vi "SerialRPC.vi"(8 "error in (no error)":errorcluster, 9 "Timeout":dbl=10000.0, 10 "Serial Port":refnum<visa-resource-name>="COM5", 11 "Baud Rate":u32=9600) -> (0 "error out":errorcluster, 3 "mbed.lvclass":refnum<class "mbed.lvclass">)   [LabVIEW 2011, in "mbed_LVLibrary.lvlib" / "SerialRPC.lvclass"]
doc: "This constructs an mbed object connected over Serial port. The mbed must be running code which receives data over the USB virtual serial port and passes it to the RPC function. See the mbed cookbook for code for the mbed http://mbed.org/cookbook/Interfacing-with-LabVIEW \nPass into this the port and baud rate."
uses:
  SerialRPC.lvclass
  mbed/mbed.lvclass
  <vilib>/Instr/_visa.llb/VISA Set IO Buffer Mask.ctl
  SerialRPC.lvclass/SerialRPC.ctl
  <vilib>/Instr/_visa.llb/VISA Configure Serial Port (Instr).vi
panel:
  in  "mbed_LVLibrary.lvlib:SerialRPC.lvclass":refnum<class "SerialRPC.lvclass">
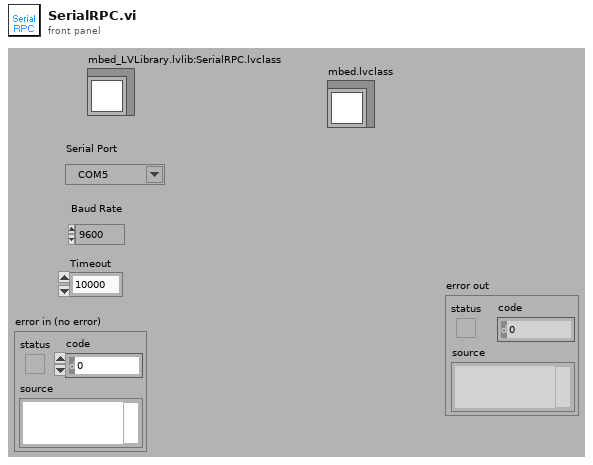
[diagram p1: front panel]
types:
  T1 = typedef "VISA Set IO Buffer Mask.ctl" = u16
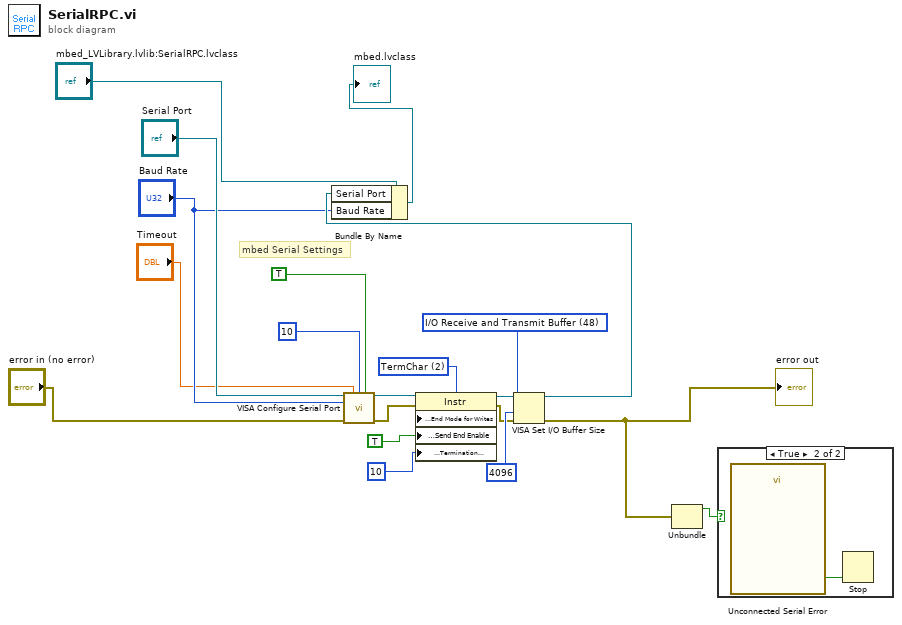
[diagram p0: block diagram]
diagram:
  w11 = T1 48 items=["I/O Receive Buffer"=16, "I/O Transmit Buffer"=32, "I/O Receive and Transmit Buffer"=48] ("Mask")
  w17 = u16 2 items=["None", "Last Bit", "TermChar", "Break"] ("Serial Settings:End Mode for Writes")
  # "mbed Serial Settings"
  n1 = call-poly "VISA Configure Serial Port"("VISA resource name"="Serial Port", "timeout (10sec)"="Timeout", "termination char\n(0xA = '\\n' = LF)"=u8 10 ("termination char\n(0xA = '\\n' = LF)"), "Enable Termination\nChar (T)"=TRUE ("Enable Termination\nChar (T)"), "baud rate (9600)"="Baud Rate", "error in (no error)"="error in (no error)") -> ("VISA resource name out"=w16:refnum<visa-resource-name>, "error out"=w14:errorcluster)  [unwired: 8 in]
  n2 = property class="Instr"(reference=w16, error in=w14, "Serial Settings:End Mode for Writes"=w17, "Message Based Settings:Send End Enable"=TRUE, "Message Based Settings:Termination Character"=u8 10) -> (reference out=w15:refnum<visa-resource-name>, error out=w13:errorcluster)
  n3 = VISA Set I/O Buffer Size(VISA resource name=w15, mask (16)=w11, size (4096)=u32 4096, error in (no error)=w13) -> (VISA resource name out=w9:refnum<visa-resource-name>, error out=w2:errorcluster)
  "error out" <- w2
  n4 = Bundle By Name(cluster="mbed_LVLibrary.lvlib:SerialRPC.lvclass", "Serial Port"=w9, "Baud Rate"="Baud Rate") -> (→"mbed.lvclass":refnum<class "SerialRPC.lvclass">)
  n5 = Unbundle(w2) -> ("status"=w3:bool)  [unwired: 2 out]
  n6 = case shown="True" w3 {
    frame False {
    }
    frame True {
      n7 = call "Unconnected Serial Error"() -> ("OK"=w21:bool)  [unwired: 10 in, 1 out]
      n8 = Stop(stop? (T)=w21) -> ()
    }
  }
